vi "Convert Ecliptic to Equatorial.vi"(0 "Epsilon":dbl=23.44014133542867 format="%.6f", 1 "Lambda":dbl=199.9060645627208 format="%.6f", 3 "Beta":dbl=0.00019384554257386913 format="%.6f") -> (4 "RA (h:m:s)":string="13:13:30.766", 5 "DEC (d:m:s)":string="-7:47:1.865", 7 "Right Ascension (alpha) in degrees":dbl=198.37819040436275 format="%.6f", 8 "Declination (delta) in degrees":dbl=-7.783851453014914 format="%.6f")   [LabVIEW 2015]
doc: "This VI calculates a general coordinate system conversion using the methods described in \"Practical Astronomy With Your Calculator\" 3rd Edition, by Peter Duffett-Smith (1988)."
panel:
  out "atan2(x,y)":dbl=-2.820832720475235 format="%.2f"
  out "y":dbl=-0.31238277949366167 format="%.2f"
  out "x":dbl=-0.9402520937294941 format="%.2f"
  # "This VI calculatesconverts ecliptic longitude (lambda) and ecliptic latitude (beta) into\nright ascension (alpha) and declination (delta)  using the methods described in Section 27 (page 40) of\n\"Practical Astronomy With Your Calculator\" 3rd Edition, by Peter Duffett-Smith (1988).\n\nThe only difference is that here we use an arctan function called Inverse Tangent (2 input) which\nautomatically removes the ambiguity and works in all quadrants of the xy plane."
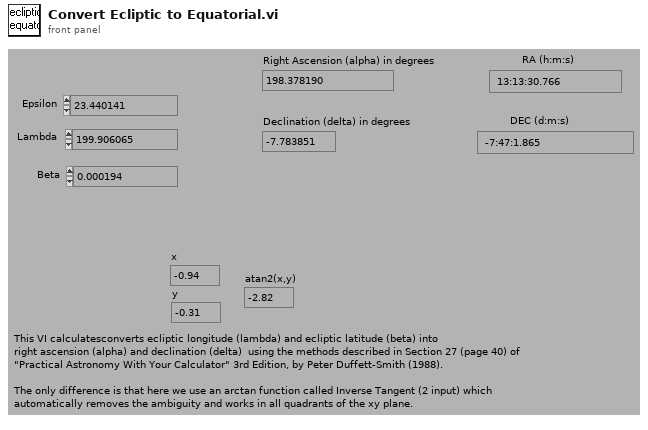
[diagram p1: front panel]
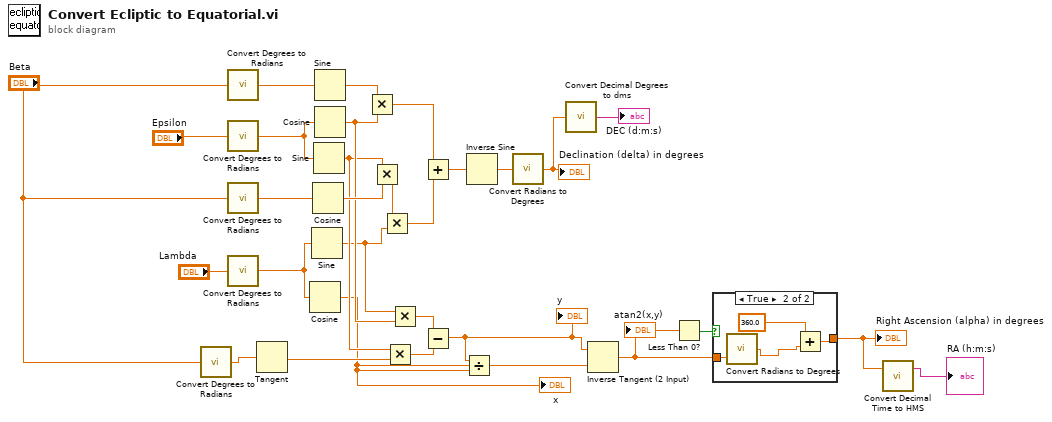
[diagram p0: block diagram]
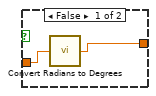
[diagram p2: hidden frame]
diagram:
  n1 = call "Convert Degrees to Radians.vi"("degrees"="Beta") -> ("radians"=w7:dbl)
  n2 = call "Convert Degrees to Radians.vi"("degrees"="Beta") -> ("radians"=w23:dbl)
  n3 = call "Convert Degrees to Radians.vi"("degrees"="Epsilon") -> ("radians"=w22:dbl)
  n4 = call "Convert Degrees to Radians.vi"("degrees"="Beta") -> ("radians"=w21:dbl)
  n5 = call "Convert Degrees to Radians.vi"("degrees"="Lambda") -> ("radians"=w15:dbl)
  n6 = Tangent(1:w7) -> (0:w10:dbl)
  n7 = Cosine(x=w15) -> (cos(x)=w5:dbl)
  "x" <- w5
  n8 = Sine(x=w15) -> (sin(x)=w9:dbl)
  n9 = Cosine(x=w21) -> (cos(x)=w28:dbl)
  n10 = Sine(x=w22) -> (sin(x)=w18:dbl)
  n11 = Sine(x=w23) -> (sin(x)=w11:dbl)
  n12 = Cosine(x=w22) -> (cos(x)=w19:dbl)
  n13 = Multiply(x=w11, y=w19) -> (x*y=w25:dbl)
  n14 = Multiply(x=w18, y=w28) -> (x*y=w27:dbl)
  n15 = Multiply(x=w27, y=w9) -> (x*y=w26:dbl)
  n16 = Multiply(x=w18, y=w10) -> (x*y=w16:dbl)
  n17 = Multiply(x=w9, y=w19) -> (x*y=w17:dbl)
  n18 = Add(x=w25, y=w26) -> (x+y=w20:dbl)
  n19 = Subtract(x=w17, y=w16) -> (x-y=w6:dbl)
  "y" <- w6
  n20 = Divide(x=w6, y=w5) -> ()  [unwired: 1 out]
  n21 = Inverse Sine(1:w20) -> (0:w24:dbl)
  n22 = call "Convert Radians to Degrees.vi"("radians"=w24) -> ("degrees"=w12:dbl)
  "Declination (delta) in degrees" <- w12
  n23 = call "Convert Decimal Degrees to dms.vi"("Decimal Degrees"=w12) -> ("Deg:Min:Sec"=→"DEC (d:m:s)":string)
  n24 = Inverse Tangent (2 Input)(1:w5, 2:w6) -> (0:w3:dbl)
  "atan2(x,y)" <- w3
  n25 = Less Than 0?(x=w3) -> (x < 0?=w4:bool)
  n26 = case shown="True" w4 {
    tunnel: w3 -> [w31 w35]
    tunnel: [w30 w33] -> w2
    frame False {
      n27 = call "Convert Radians to Degrees.vi"("radians"=w31) -> ("degrees"=w30:dbl)
    }
    frame True {
      n28 = call "Convert Radians to Degrees.vi"("radians"=w35) -> ("degrees"=w32:dbl)
      n29 = Add(x=360.0, y=w32) -> (x+y=w33:dbl)
    }
  }
  "Right Ascension (alpha) in degrees" <- w2
  n30 = call "Convert Decimal Time to HMS.vi"("Decimal Time"=w2) -> ("HMS Time"=→"RA (h:m:s)":string)  [unwired: 2 out]
